vi "Steering output parameters.vi"   [LabVIEW 2016]
uses:
  Robot Global Data.vi
types:
  T1 = enum16{"min count rotation", "max count rotation ", "offset count to zero wheel"}
  T2 = enum16{"FL Drive Wheel", "FR Drive Wheel", "RL Drive Wheel", "RR Drive Wheel", "FL Steer Wheel", "FR Steer Wheel", "RL Steer Wheel", "RR Steer Wheel"}
  T3 = typedef "WPI_MotorControlDeviceRef.ctl" = cluster{"DeviceStatus":errorcluster, "Type":T4, "PWM":cluster{"PWM Channel":T5, "DeadBand":T6}, "CAN":cluster{"Device Number":u8, "SetOutput VI Ref":variant, "GetOutput VI Ref":variant, "Enable VI Ref":variant, "Disable VI Ref":variant, "Data":variant}, "Invert":bool}
  T4 = typedef "WPI_MotorControlType.ctl" = enum16{"PWM", "CAN"}
  T5 = typedef "FPGA_DIOPWMChannel.ctl" = enum8{"PWM 0", "PWM 1", "PWM 2", "PWM 3", "PWM 4", "PWM 5", "PWM 6", "PWM 7", "PWM 8", "PWM 9", "PWM MXP 0", "PWM MXP 1", "PWM MXP 2", "PWM MXP 3", "PWM MXP 4", "PWM MXP 5", "PWM MXP 6", "PWM MXP 7", "PWM MXP 8", "PWM MXP 9", "Invalid"}
  T6 = typedef "WPI_PWMDeadband.ctl" = cluster{"Name":string, "maxPositivePwm":i32, "minPositivePwm":i32, "centerPwm":i32, "maxNegativePwm":i32, "minNegativePwm":i32, "angularRange":u16}
  T7 = typedef "WPI_CANTalonSRX_GlobalStatus.ctl" = cluster{"Applied Throttle":dbl, "Module Enabled":bool, "CAN Error":errorcluster, "Closed Loop Error":dbl, "Forward Limit Switch Closed":bool, "Reverse Limit Switch Closed":bool, "Sensor Position":dbl, "Sensor Velocity":dbl, "Current":dbl, "Sticky Fault - Over Temp":bool, "Sticky Fault - Under Voltage":bool, "Sticky Fault - Forward Limit":bool, "Sticky Fault - Reverse Limit":bool, "Sticky Fault - Forward Soft Limit":bool, "Sticky Fault - Reverse Soft Limit":bool, "Brake is Enabled":bool, "Encoder Position":dbl, "Encoder Velocity":dbl, "Encoder Index Count":dbl, "Encoder A Pin State":bool, "Encoder B Pin State":bool, "Encoder Index Pin State":bool, "Analog In":dbl, "Analog In Velocity":dbl, "Temperature (C)":dbl, "Battery Voltage":dbl, "Control 5 Is Supported":bool, "Current Profile Slot Select":dbl, "Pos Div 8":bool, "Vel Div 4":bool, "Pulse Width Position":i32, "Pulse Width Velocity":i32, "Pulse Width Rise To Rise (us)":i32, "Pulse Width Rise To Fall (us)":i32, "Mot Prof Active Is Under Run":bool, "Mot Prof Active Has Under Run":bool, "Mot Prof Active Is Last":bool, "Mot Prof Active Velocity Only":bool, "Mot Prof Active Is Valid":bool, "Mot Prof Buffer Is Full":bool, "Mot Prof Active Profile Slot Select":i32, "Mot Prof NextID":i32, "Mot Prof Count":i32, "Mot Prof Active Velocity":dbl, "Mot Prof Active Position":dbl, "Mot Prof Output Enable":i32}
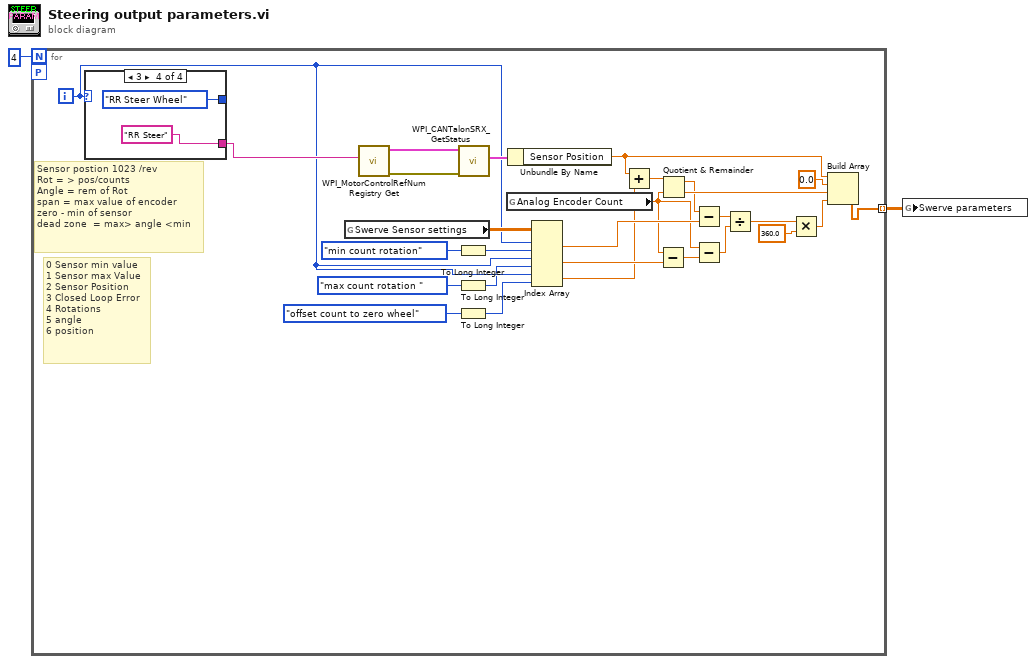
[diagram p0: block diagram]
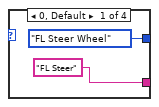
[diagram p2: hidden frame]
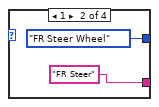
[diagram p3: hidden frame]
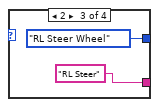
[diagram p4: hidden frame]
diagram:
  n1 = for {
    N: 4 -> [_]
    tunnel: [w15] -> w1 mode=indexing
    workers-P: _ -> [_]
    i -> [w12]
    # "0 Sensor min value\n1 Sensor max Value\n2 Sensor Position\n3 Closed Loop Error\n4 Rotations\n5 angle\n6 position"
    # "Sensor postion 1023 /rev\nRot = > pos/counts\nAngle = rem of Rot\nspan = max value of encoder\nzero - min of sensor\ndead zone  = max> angle <min"
    n2 = case shown="3" w12 {
      tunnel: [T2."FL Steer Wheel" ("Swerve Drive Param") T2."FR Steer Wheel" ("Swerve Drive Param") T2."RL Steer Wheel" ("Swerve Drive Param") T2."RR Steer Wheel" ("Swerve Drive Param")] -> _
      tunnel: ["FL Steer" ("refnum name") "FR Steer" ("refnum name") "RL Steer" ("refnum name") "RR Steer" ("refnum name")] -> w16
      frame 0, Default {
      }
      frame 1 {
      }
      frame 2 {
      }
      frame 3 {
      }
    }
    n3 = global read "Robot Global Data.vi" "Swerve Sensor settings"() -> (w25:dbl[][])
    n4 = call <vilib>:"WPI_MotorControlRefNum Registry Get.vi"("refnum name"=w16) -> ("error out"=w28:errorcluster, "MotorControlDevRef"=w29:T3)  [unwired: 9 in]
    n5 = To Long Integer(number=T1."min count rotation" ("Enum")) -> (32bit integer=w6:i32)
    n6 = To Long Integer(number=T1."max count rotation " ("Enum")) -> (32bit integer=w7:i32)
    n7 = To Long Integer(number=T1."offset count to zero wheel" ("Enum")) -> (32bit integer=w8:i32)
    n8 = call <vilib>:"WPI_CANTalonSRX_GetStatus.vi"("error in (no error)"=w28, "CAN Talon SRX Ref"=w29) -> ("Talon SRX Status"=w30:T7)  [unwired: 7 in, 2 out]
    n9 = global read "Robot Global Data.vi" "Analog Encoder Count"() -> (w18:dbl)
    n10 = Unbundle By Name(w30) -> ("Sensor Position"=w4:dbl)
    n11 = Index Array(array=w25, index (row) #1=w12, index (col) #1=w6, index (row) #2=w12, index (col) #2=w7, index (row) #3=w12, index (col) #3=w8) -> (element #1=w26:dbl, element #2=w20:dbl, element #3=w3:dbl)
    n12 = Add(x=w4, y=w3) -> (x+y=w5:dbl)
    n13 = Subtract(x=w18, y=w20) -> (x-y=w19:dbl)
    n14 = Quotient & Remainder(x=w5, y=w18) -> (x-y*floor(x/y)=w23:dbl, floor(x/y)=w24:dbl)
    n15 = Subtract(x=w23, y=w26) -> (x-y=w22:dbl)
    n16 = Subtract(x=w18, y=w19) -> (x-y=w17:dbl)
    n17 = Divide(x=w22, y=w17) -> (x/y=w21:dbl)
    n18 = Multiply(x=w21, y=360.0 ("x")) -> (x*y=w14:dbl)
    n19 = Build Array(w4, 0.0 ("element"), w24, w14) -> (w15:dbl[])
  }
  n20 = global write "Robot Global Data.vi" "Swerve parameters"(w1) -> ()
